vi "Do.vi"(8 "error in (no error)":errorcluster, 10 "Actor in":refnum<class "Actor.lvclass">, 11 "4503 Actor Msg":refnum<class "4503 Actor Msg.lvclass">) -> (0 "error out":errorcluster, 2 "Actor out":refnum<class "Actor.lvclass">)   [LabVIEW 2024, in "4503 Actor.lvlib" / "4503 Actor Msg.lvclass"]
doc: "(<B>Filename</B>: Actor Framework.lvlib:Message.lvclass:Do.vi)\n\nDefines what a message does when it is received by an actor. Generally, a message instructs an actor to invoke one of its methods. By default, this method does nothing. A child class must override it to define behavior. Create a child class by using the Actor Framework Message Maker dialog box."
uses:
  4503 Actor Msg.lvclass
  <vilib>/ActorFramework/Actor/Actor.lvclass
  4503/4503.lvclass
  C:/Program Files (x86)/National Instruments/LabVIEW 2024/vi.lib/ActorFramework/Actor/Actor.lvclass
  4503 Actor Msg.lvclass/4503 Actor Msg.ctl
  <vilib>/ActorFramework/Message/Message.lvclass
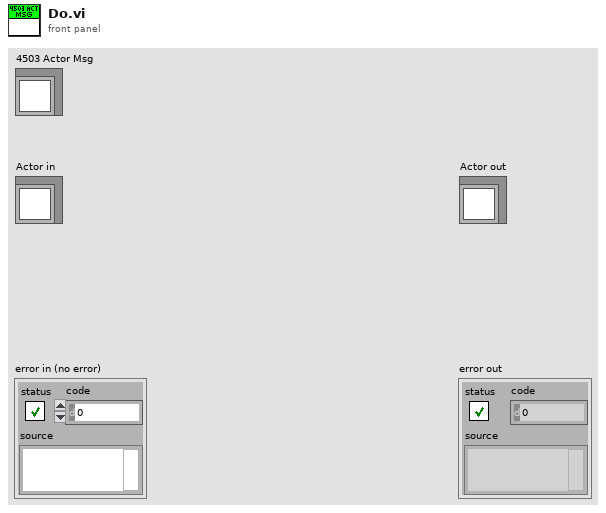
[diagram p1: front panel]
types:
  T1 = typedef "4503MsgFunc.ctl" = enum16{"StartQuery", "StopQuery", "ZeroAngle", "ClearData"}
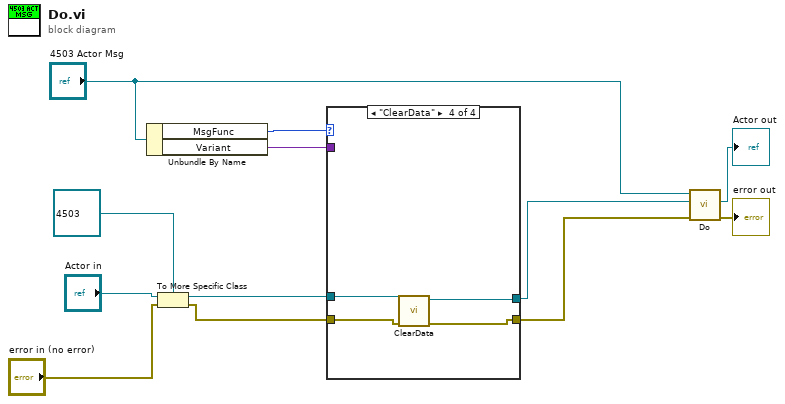
[diagram p0: block diagram]
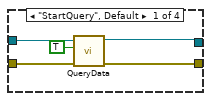
[diagram p2: hidden frame]
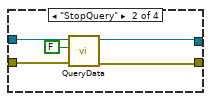
[diagram p3: hidden frame]
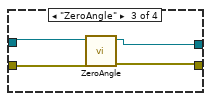
[diagram p4: hidden frame]
diagram:
  n1 = Unbundle By Name("4503 Actor Msg") -> ("MsgFunc"=w9:T1, "Variant"=w8:variant)
  n2 = To More Specific Class(target class=refnum<class "4503.lvclass"> refnum ("4503 Actor.lvlib:4503.lvclass"), reference="Actor in", error in="error in (no error)") -> (specific class reference=w4:refnum<class "4503.lvclass">, error out=w3:errorcluster)
  n3 = case shown="\"ClearData\"" w9 {
    tunnel: w8 -> [_ _ _ _]
    tunnel: w4 -> [w17 w22 w26 w30]
    tunnel: w3 -> [w15 w18 w25 w29]
    tunnel: [w14 w20 w24 w28] -> w2
    tunnel: [w13 w19 w23 w27] -> w1
    frame "StartQuery", Default {
      n4 = call "QueryData.vi"("error in (no error)"=w15, "Boolean"=TRUE, "4503 in"=w17) -> ("error out"=w13:errorcluster, "4503 out"=w14:refnum<class "4503.lvclass">)  [unwired: 7 in]
    }
    frame "StopQuery" {
      n5 = call "QueryData.vi"("error in (no error)"=w18, "Boolean"=FALSE, "4503 in"=w22) -> ("error out"=w19:errorcluster, "4503 out"=w20:refnum<class "4503.lvclass">)  [unwired: 7 in]
    }
    frame "ZeroAngle" {
      n6 = call "ZeroAngle.vi"("error in (no error)"=w25, "4503 in"=w26) -> ("error out"=w23:errorcluster, "4503 out"=w24:refnum<class "4503.lvclass">)  [unwired: 8 in]
    }
    frame "ClearData" {
      n7 = call "ClearData.vi"("error in (no error)"=w29, "4503 in"=w30) -> ("error out"=w27:errorcluster, "4503 out"=w28:refnum<class "4503.lvclass">)  [unwired: 8 in]
    }
  }
  n8 = call-parent "Do.vi"("error in (no error)"=w1, "Actor in"=w2, "Message"="4503 Actor Msg") -> ("error out"=→"error out":errorcluster, "Actor out"=→"Actor out":refnum<class "Actor.lvclass">)  [unwired: 7 in]
